vi "CVOpenCorrection.vi"(6 "Input parameters":T1={"Measurement type"=enum."Debug", "Sensor type"=enum."HPK_8in_256", "Identifier"="test.txt", "Open after execution?"=FALSE, "Plot after execution?"=FALSE, "Display channel"=0, "Voltage Delay (s)"=0.5, "Switch Delay (s)"=0.01, "VISA resource name source"="", "VISA resource name DMM"="", "VISA resource name LCR"="", "Compliance  Level (A)"=10.0, "Voltage Limit (V)"=1000.0, "Data storage location"="", "Scan voltages"="", "Use source as DMM?"=FALSE, "LCR signal frequenzy (Hz)"=10.0, "DMM device"=enum."Keithley2001", "Sampling number"=1, "Use env. sensors on"=enum."Sensirion sht1x/7x", "Switchboard Handle"=0, "Use Switchboard"=FALSE, "LCR signal voltage (V)"=10000.0, "Repeat"=1, "Scan voltages IV"="", "Scan voltages CV"="", "Hex pad numbers?"=FALSE, "Set measurement type"=enum."Debug", "Custom pad scan"="", "IV voltage Delay (s)"=0.5, "CV voltage Delay (s)"=0.5, "Needle measurement?"=FALSE, "Comments"="test.txt", "LCR signal frequenzy (kHz)"=10.0, "Compliance  Level (uA)"=10.0, "Open Correction Array"=array2304x3[6912 elements], "Current set voltage"=0.0, "Last set voltage"=0.0, "Current channel"=0, "Last OpenCorrection index"=-1, "Total curr/vltg every x steps"=10, "Current channel iteration"=0, "No CV corrections"=FALSE} {"Last set voltage" format="%#_13g"; "Current set voltage" format="%#_13g"; "CV voltage Delay (s)" format="%#_13g"; "IV voltage Delay (s)" format="%#_13g"; "Voltage Limit (V)" format="%#_13g"; "Voltage Delay (s)" format="%#_13g"; "Switch Delay (s)" format="%#_13g"}, 8 "error in (no error)":errorcluster, 10 "Cs [pF]":dbl=100.0, 11 "Cp [pF]":dbl=100.0) -> (0 "error out":errorcluster, 1 "Cs corrected [pF]":dbl=10000.0, 2 "Cp corrected [pF]":dbl=10000.0, 3 "Input parameters out":T1={"Measurement type"=enum."Debug", "Sensor type"=enum."HPK_8in_256", "Identifier"="test.txt", "Open after execution?"=FALSE, "Plot after execution?"=FALSE, "Display channel"=0, "Voltage Delay (s)"=0.5, "Switch Delay (s)"=0.01, "VISA resource name source"="", "VISA resource name DMM"="", "VISA resource name LCR"="", "Compliance  Level (A)"=10.0, "Voltage Limit (V)"=1000.0, "Data storage location"="", "Scan voltages"="", "Use source as DMM?"=FALSE, "LCR signal frequenzy (Hz)"=10.0, "DMM device"=enum."Keithley2001", "Sampling number"=1, "Use env. sensors on"=enum."Sensirion sht1x/7x", "Switchboard Handle"=0, "Use Switchboard"=FALSE, "LCR signal voltage (V)"=10000.0, "Repeat"=1, "Scan voltages IV"="", "Scan voltages CV"="", "Hex pad numbers?"=FALSE, "Set measurement type"=enum."Debug", "Custom pad scan"="", "IV voltage Delay (s)"=0.5, "CV voltage Delay (s)"=0.5, "Needle measurement?"=FALSE, "Comments"="test.txt", "LCR signal frequenzy (kHz)"=10.0, "Compliance  Level (uA)"=10.0, "Open Correction Array"=array2304x3[6912 elements], "Current set voltage"=0.0, "Last set voltage"=0.0, "Current channel"=0, "Last OpenCorrection index"=-1, "Total curr/vltg every x steps"=10, "Current channel iteration"=0, "No CV corrections"=FALSE} {"Last set voltage" format="%#_13g"; "Current set voltage" format="%#_13g"; "CV voltage Delay (s)" format="%#_13g"; "IV voltage Delay (s)" format="%#_13g"; "Voltage Limit (V)" format="%#_13g"; "Voltage Delay (s)" format="%#_13g"; "Switch Delay (s)" format="%#_13g"})   [LabVIEW 2016]
uses:
  Input_parameters.ctl
panel:
  out "Last set voltage":dbl
  out "Current set voltage":dbl
  out "Open Correction Array":dbl[][](array[numeric])
  out "C_p_open at current voltage and channel":dbl
  out "Next occurance of current channel":i32
  out "First occurance of current voltage":i32
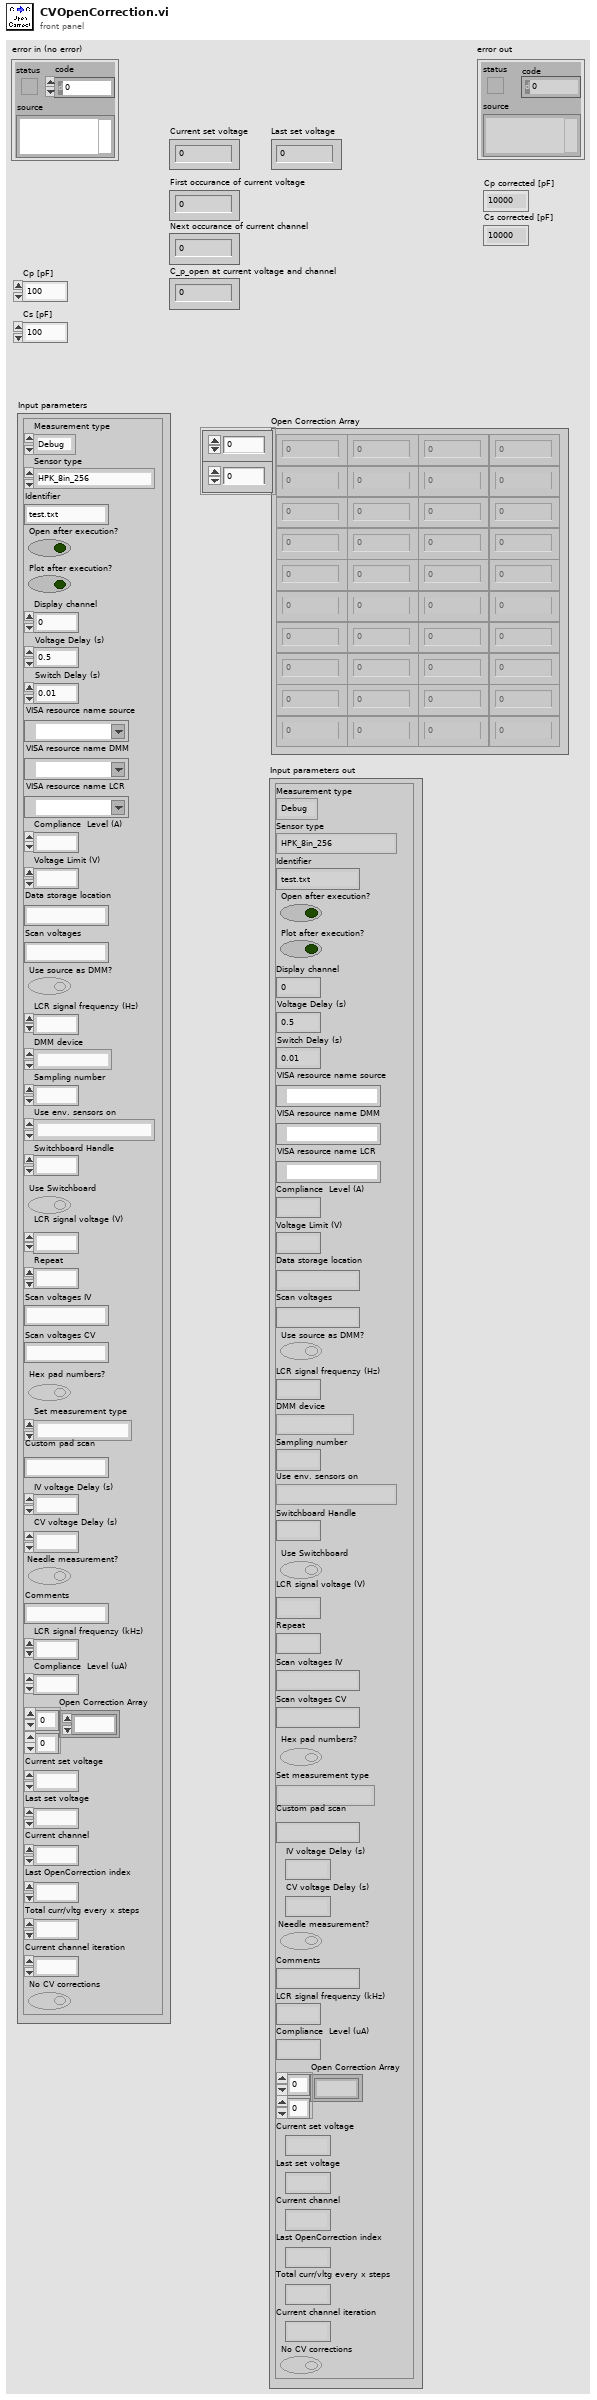
[diagram p1: front panel]
types:
  T1 = typedef "Input_parameters.ctl" = cluster{"Measurement type":enum16{"IV", "CV", "Debug", "Test_contact"}, "Sensor type":enum16{"HPK_6in_135", "HPK_8in_256", "IFX_8in_256", "Diode", "HPK_6in_256", "Test capacitances", "Full matrix"}, "Identifier":string, "Open after execution?":bool, "Plot after execution?":bool, "Display channel":i32, "Voltage Delay (s)":dbl, "Switch Delay (s)":dbl, "VISA resource name source":refnum<visa-resource-name>, "VISA resource name DMM":refnum<visa-resource-name>, "VISA resource name LCR":refnum<visa-resource-name>, "Compliance  Level (A)":dbl, "Voltage Limit (V)":dbl, "Data storage location":string, "Scan voltages":string, "Use source as DMM?":bool, "LCR signal frequenzy (Hz)":dbl, "DMM device":enum16{"Keithley2001", "Keithley2450", "Keithley2410", "Keithley6487"}, "Sampling number":i32, "Use env. sensors on":enum16{"Sensirion sht1x/7x", "Switch Matrix", "Probecard"}, "Switchboard Handle":u32, "Use Switchboard":bool, "LCR signal voltage (V)":dbl, "Repeat":i32, "Scan voltages IV":string, "Scan voltages CV":string, "Hex pad numbers?":bool, "Set measurement type":enum16{"IV", "CV", "Debug", "Test_contact", "IV+CV"}, "Custom pad scan":string, "IV voltage Delay (s)":dbl, "CV voltage Delay (s)":dbl, "Needle measurement?":bool, "Comments":string, "LCR signal frequenzy (kHz)":dbl, "Compliance  Level (uA)":dbl, "Open Correction Array":dbl[][], "Current set voltage":dbl, "Last set voltage":dbl, "Current channel":i32, "Last OpenCorrection index":i32, "Total curr/vltg every x steps":i32, "Current channel iteration":i32, "No CV corrections":bool}
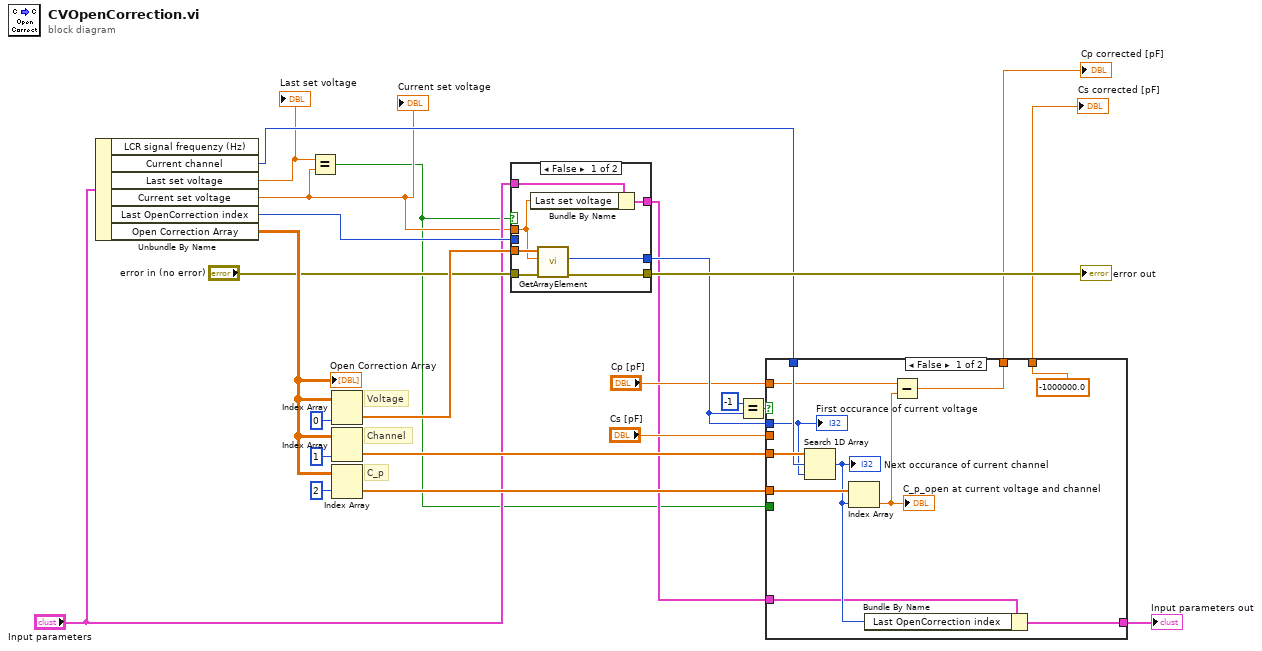
[diagram p0: block diagram]
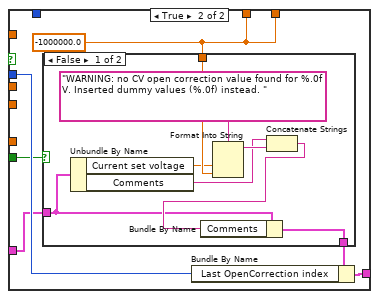
[diagram p2: hidden frame]
diagram:
  # "C_p"
  # "Voltage"
  # "Channel"
  n1 = Unbundle By Name("Input parameters") -> ("Current channel"=w15:i32, "Last set voltage"=w14:dbl, "Current set voltage"=w2:dbl, "Last OpenCorrection index"=w13:i32, "Open Correction Array"=w19:dbl[][])  [unwired: 1 out]
  "Open Correction Array" <- w19
  "Current set voltage" <- w2
  "Last set voltage" <- w14
  n2 = Equal?(x=w14, y=w2) -> (x = y?=w1:bool)
  n3 = Index Array(array=w19, index (col)=0 ("disabled index (col)")) -> (element=w18:dbl[])  [unwired: 1 in]
  n4 = Index Array(array=w19, index (col)=1 ("disabled index (col)")) -> (element=w22:dbl[])  [unwired: 1 in]
  n5 = Index Array(array=w19, index (col)=2 ("disabled index (col)")) -> (element=w20:dbl[])  [unwired: 1 in]
  n6 = case shown="False" w1 {
    tunnel: w18 -> [w31 _]
    tunnel: [w30 w34] -> w11
    tunnel: "error in (no error)" -> [w29 w33]
    tunnel: [w28 w33] -> w16
    tunnel: w2 -> [w25 _]
    tunnel: w13 -> [_ w34]
    tunnel: "Input parameters" -> [w26 w32]
    tunnel: [w27 w32] -> w4
    frame False {
      n7 = Bundle By Name(cluster=w26, "Last set voltage"=w25) -> (w27:T1)
      n8 = call "GetArrayElement.vi"("error in (no error)"=w29, "Desired element"=w25, "Array"=w31) -> ("error out"=w28:errorcluster, "New index"=w30:i32)  [unwired: 7 in]
    }
    frame True {
    }
  }
  "error out" <- w16
  n9 = Equal?(x=-1 ("y"), y=w11) -> (x = y?=w9:bool)
  n10 = case shown="False" w9 {
    tunnel: w22 -> [w45 _]
    tunnel: w20 -> [w44 _]
    tunnel: w15 -> [w43 _]
    tunnel: w11 -> [w42 w51]
    tunnel: "Cp [pF]" -> [w40 _]
    tunnel: [w39 w49] -> w7
    tunnel: "Cs [pF]" -> [_ _]
    tunnel: [-1000000.0 ("Cs corrected [pF]") w49] -> w5
    tunnel: w4 -> [w35 w47]
    tunnel: [w36 w50] -> w3
    tunnel: w1 -> [_ w46]
    frame False {
      n11 = Search 1D Array(1D array=w45, element=w43, start index (0)=w42) -> (index of element=w37:i32)
      "Next occurance of current channel" <- w37
      n12 = Index Array(array=w44, index=w37) -> (element=w41:dbl)
      "C_p_open at current voltage and channel" <- w41
      n13 = Bundle By Name(cluster=w35, "Last OpenCorrection index"=w37) -> (w36:T1)
      n14 = Subtract(x=w40, y=w41) -> (x-y=w39:dbl)
      "First occurance of current voltage" <- w42
    }
    frame True {
      w49 = -1000000.0 ("Cs corrected [pF]")
      n15 = case shown="False" w46 {
        tunnel: w49 -> [w58 _]
        tunnel: [w53 w60] -> w48
        tunnel: w47 -> [w52 w60]
        frame False {
          n16 = Unbundle By Name(w52) -> ("Current set voltage"=w57:dbl, "Comments"=w55:string)
          n17 = Format Into String(format string="WARNING: no CV open correction value found for %.0f V. Inserted dummy values (%.0f) instead. ", w57, w58) -> (resulting string=w56:string)  [unwired: 2 in, 1 out]
          n18 = Concatenate Strings(w55, w56) -> (w54:string)
          n19 = Bundle By Name(cluster=w52, "Comments"=w54) -> (w53:T1)
        }
        frame True {
        }
      }
      n20 = Bundle By Name(cluster=w48, "Last OpenCorrection index"=w51) -> (w50:T1)
    }
  }
  "Cp corrected [pF]" <- w7
  "Cs corrected [pF]" <- w5
  "Input parameters out" <- w3
